vi "send_trigger.vi"(8 "error in (no error)":errorcluster, 10 "trigger":T1, 11 "GenericDataCollection in":refnum<class "GenericDataCollection.lvclass">) -> (0 "error out":errorcluster, 3 "GenericDataCollection out":refnum<class "GenericDataCollection.lvclass">)   [LabVIEW 2010, in "GenericDataCollection.lvclass"]
uses:
  GenericDataCollection.lvclass
  trigger_enum.ctl
  common/classes/GenericToplevelComponent/GenericToplevelComponent/trigger_type_enum.ctl
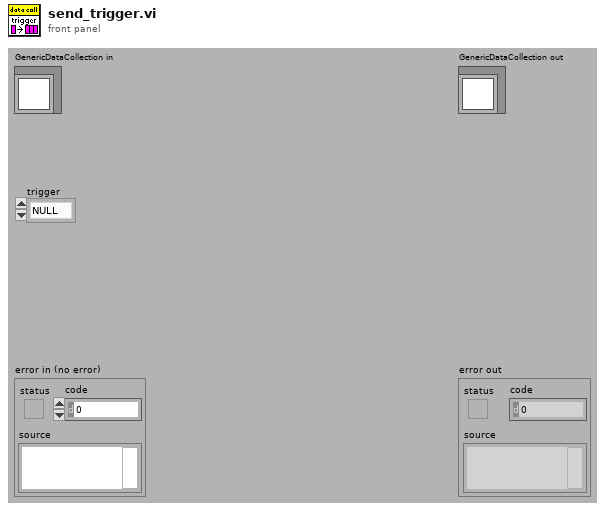
[diagram p1: front panel]
types:
  T1 = typedef "GenericDataCollection.lvclass/trigger_enum.ctl" = enum16{"NULL", "save", "reset"}
  T2 = typedef "trigger_type_enum.ctl" = enum8{"external", "internal", "common"}
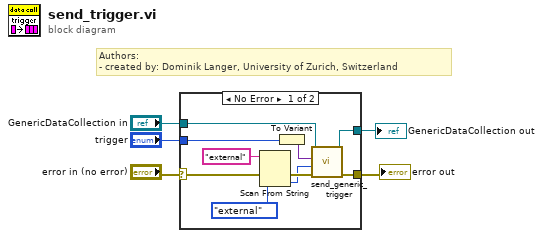
[diagram p0: block diagram]
diagram:
  # "Authors: \n- created by: Dominik Langer, University of Zurich, Switzerland"
  n1 = case shown="No Error" "error in (no error)" {
    selector: "error in (no error)" -> [w10 w17]
    tunnel: [w14 w17] -> w1
    tunnel: [w13 w16] -> w2
    tunnel: "GenericDataCollection in" -> [w11 w16]
    tunnel: "trigger" -> [w15 _]
    frame No Error {
      n2 = Scan From String(input string="external", error in=w10, default 1=trigger_type_enum."external" ("trigger type")) -> (error out=w9:errorcluster, output 1=w7:T2)  [unwired: 2 in, 2 out]
      n3 = To Variant(anything=w15) -> (Variant=w12:variant)
      n4 = call-dynamic "send_generic_trigger.vi"("error in (no error)"=w9, "trigger type"=w7, "trigger variant"=w12, "GenericToplevelComponent in"=w11) -> ("error out"=w14:errorcluster, "GenericToplevelComponent out"=w13:refnum<class "GenericDataCollection.lvclass">)  [unwired: 4 in, 2 out]
    }
    frame Error {
    }
  }
  "error out" <- w1
  "GenericDataCollection out" <- w2
